vi "CSDB_Config.apply mapping.vi"(1 "Enum":enum16{"i 2 BP", "BP 2 i", "get"}(ring), 2 "ClassName":string, 3 "AttributeNamesIn":string[](array[string]), 4 "Values in":string[][](array[string]), 5 "error in (no error)":errorcluster) -> (17 "AttributeNames out":string[](array[string]), 18 "Values out":string[][](array[string]), 19 "error out":errorcluster)   [LabVIEW 2014, in "CSDB_Config.lvlib"]
doc: "hm..."
uses:
  CSDB_Config.lvlib
  <vilib>/Utility/config.llb/Read Key (String).vi
  <vilib>/Utility/config.llb/NI_LVConfig.lvlib
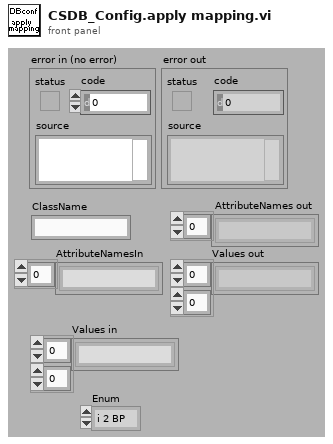
[diagram p1: front panel]
types:
  T1 = typedef "NI_LVConfig.lvlib/Config Data RefNum.ctl" = refnum<k1>
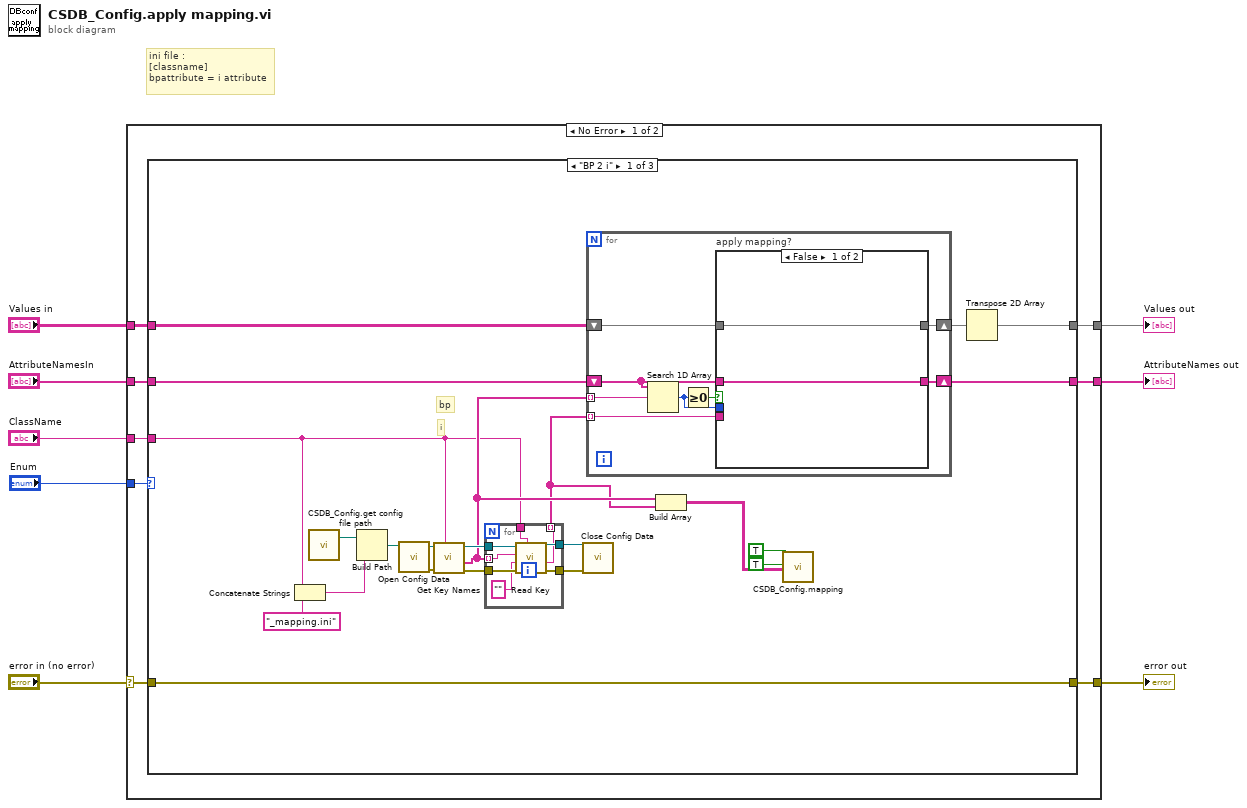
[diagram p0: block diagram]
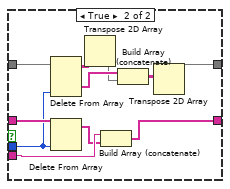
[diagram p2: hidden frame]
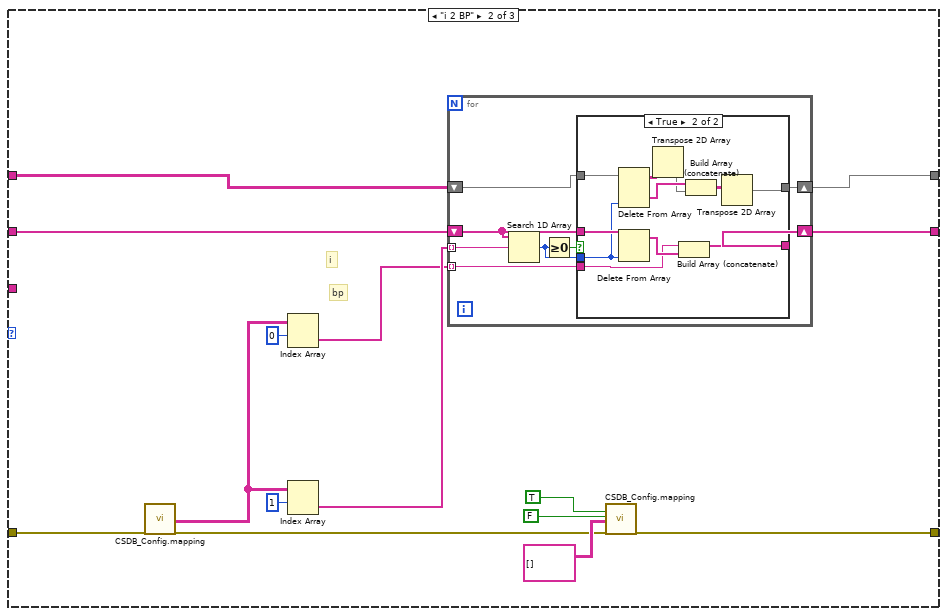
[diagram p3: hidden frame]
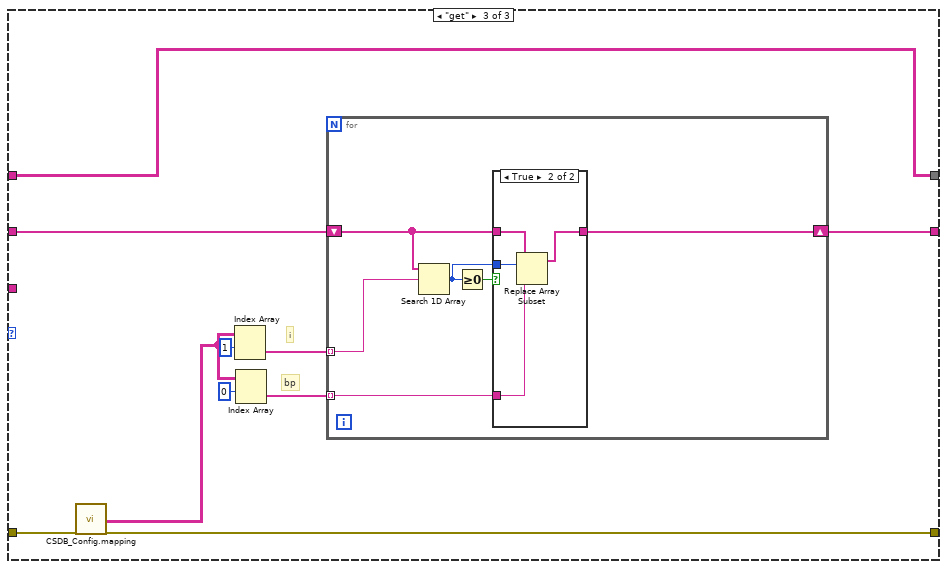
[diagram p5: hidden frame]
diagram:
  # "ini file :\n[classname]\nbpattribute = i attribute"
  n1 = case shown="No Error" "error in (no error)" {
    selector: "error in (no error)" -> [w9 w127]
    tunnel: [w16 w127] -> w8
    tunnel: "ClassName" -> [w15 _]
    tunnel: "AttributeNamesIn" -> [w14 w125]
    tunnel: [w13 w125] -> w5
    tunnel: "Values in" -> [w12 w126]
    tunnel: [w11 w126] -> w3
    tunnel: "Enum" -> [w10 _]
    frame No Error {
      n2 = case shown="\"BP 2 i\"" w10 {
        tunnel: w9 -> [w38 w77 w106]
        tunnel: [w38 w82 w105] -> w16
        tunnel: w15 -> [w18 _ _]
        tunnel: w14 -> [w37 w81 w113]
        tunnel: [w36 w80 w112] -> w13
        tunnel: w12 -> [w35 w79 w111]
        tunnel: [w34 w78 w111] -> w11
        frame "BP 2 i" {
          # "i"
          # "bp"
          n3 = Concatenate Strings(w18, "_mapping.ini" ("name or relative path")) -> (w17:string)
          n4 = call "CSDB_Config.get config file path.vi"() -> ("config file path"=w23:path)  [unwired: 18 in, 1 out]
          n5 = Build Path(base path=w23, name or relative path=w17) -> (appended path=w24:path)
          n6 = call <vilib>:"Open Config Data.vi"("configuration file path"=w24) -> ("error out"=w31:errorcluster, "refnum"=w32:T1)  [unwired: 8 in, 1 out]
          n7 = call <vilib>:"Get Key Names.vi"("section"=w18, "error in (no error)"=w31, "refnum"=w32) -> ("error out"=w29:errorcluster, "key names"=w26:string[], "refnum out"=w30:T1)  [unwired: 5 in, 1 out]
          n8 = for {
            tunnel: w30 -> [w67]
            tunnel: w29 -> [w62]
            tunnel: w18 -> [w66]
            tunnel: w26 -> [w65] mode=indexing
            tunnel: [w64] -> w28
            tunnel: [w63] -> w27
            tunnel: [w60] -> w25 mode=indexing
            n9 = call-poly <vilib>:"Read Key.vi"("section"=w66, "error in (no error)"=w62, "default value"="", "key"=w65, "refnum"=w67) -> ("error out"=w63:errorcluster, "value"=w60:string, "refnum out"=w64:T1)  [unwired: 3 in, 1 out]
          }
          n10 = call <vilib>:"Close Config Data.vi"("error in (no error)"=w27, "refnum"=w28) -> ()  [unwired: 8 in, 2 out]
          n11 = for {
            tunnel: w26 -> [w41] mode=indexing
            tunnel: w25 -> [w42] mode=indexing
            shift-right: [w43] -> w36
            shift-left: w37 -> [w45]
            shift-right: [w39] -> w33
            shift-left: w35 -> [w40]
            n12 = Search 1D Array(1D array=w45, element=w41) -> (index of element=w44:i32)  [unwired: 1 in]
            n13 = Greater Or Equal To 0?(x=w44) -> (x >= 0?=w46:bool)
            n14 = case "apply mapping?" shown="False" w46 {
              tunnel: w45 -> [w48 w59]
              tunnel: w44 -> [_ w56]
              tunnel: w42 -> [_ w54]
              tunnel: [w48 w58] -> w43
              tunnel: w40 -> [w47 w57]
              tunnel: [w47 w55] -> w39
              frame False {
              }
              frame True {
                n15 = Delete From Array(array=w57, index (col)=w56) -> (deleted portion=w52:string[], array with subset deleted=w50:string[][])  [unwired: 2 in]
                n16 = Delete From Array(array=w59, index=w56) -> (array with subset deleted=w53:string[])  [unwired: 1 in, 1 out]
                n17 = Transpose 2D Array(2D array=w50) -> (transposed array=w49:string[][])
                n18 = Build Array (concatenate)(w54, w53) -> (w58:string[])
                n19 = Build Array (concatenate)(w52, w49) -> (w51:string[][])
                n20 = Transpose 2D Array(2D array=w51) -> (transposed array=w55:string[][])
              }
            }
          }
          n21 = Build Array(w26, w25) -> (w22:string[][])
          n22 = call "CSDB_Config.mapping.vi"("setMapping"=TRUE, "useMapping"=TRUE, "mapping"=w22) -> ()  [unwired: 14 in, 3 out]
          n23 = Transpose 2D Array(2D array=w33) -> (transposed array=w34:string[][])
        }
        frame "i 2 BP" {
          # "i"
          # "bp"
          n24 = call "CSDB_Config.mapping.vi"("error in (no error)"=w77) -> ("mapping out"=w71:string[][], "error out"=w70:errorcluster)  [unwired: 16 in, 1 out]
          n25 = Index Array(array=w71, index (row)=0) -> (element=w73:string[])  [unwired: 1 in]
          n26 = Index Array(array=w71, index (row)=1) -> (element=w74:string[])  [unwired: 1 in]
          n27 = for {
            tunnel: w74 -> [w85] mode=indexing
            tunnel: w73 -> [w86] mode=indexing
            shift-right: [w87] -> w80
            shift-left: w81 -> [w89]
            shift-right: [w83] -> w78
            shift-left: w79 -> [w84]
            n28 = Search 1D Array(1D array=w89, element=w85) -> (index of element=w88:i32)  [unwired: 1 in]
            n29 = Greater Or Equal To 0?(x=w88) -> (x >= 0?=w90:bool)
            n30 = case shown="True" w90 {
              tunnel: w89 -> [w92 w103]
              tunnel: w88 -> [_ w97]
              tunnel: w86 -> [_ w100]
              tunnel: [w92 w102] -> w87
              tunnel: w84 -> [w91 w99]
              tunnel: [w91 w95] -> w83
              frame False {
              }
              frame True {
                n31 = Delete From Array(array=w99, index (col)=w97) -> (deleted portion=w98:string[], array with subset deleted=w94:string[][])  [unwired: 2 in]
                n32 = Delete From Array(array=w103, index=w97) -> (array with subset deleted=w101:string[])  [unwired: 1 in, 1 out]
                n33 = Transpose 2D Array(2D array=w94) -> (transposed array=w93:string[][])
                n34 = Build Array (concatenate)(w100, w101) -> (w102:string[])
                n35 = Build Array (concatenate)(w98, w93) -> (w96:string[][])
                n36 = Transpose 2D Array(2D array=w96) -> (transposed array=w95:string[][])
              }
            }
          }
          n37 = call "CSDB_Config.mapping.vi"("setMapping"=TRUE, "useMapping"=FALSE, "mapping"=string[][] [], "error in (no error)"=w70) -> ("error out"=w82:errorcluster)  [unwired: 13 in, 2 out]
        }
        frame "get" {
          # "i"
          # "bp"
          n38 = call "CSDB_Config.mapping.vi"("error in (no error)"=w106) -> ("mapping out"=w104:string[][], "error out"=w105:errorcluster)  [unwired: 16 in, 1 out]
          n39 = Index Array(array=w104, index (row)=1 ("disabled index (col)")) -> (element=w110:string[])  [unwired: 1 in]
          n40 = Index Array(array=w104, index (row)=0 ("disabled index (col)")) -> (element=w107:string[])  [unwired: 1 in]
          n41 = for {
            tunnel: w110 -> [w119] mode=indexing
            tunnel: w107 -> [w115] mode=indexing
            shift-right: [w114] -> w112
            shift-left: w113 -> [w117]
            n42 = Search 1D Array(1D array=w117, element=w119) -> (index of element=w116:i32)  [unwired: 1 in]
            n43 = Greater Or Equal To 0?(x=w116) -> (x >= 0?=w118:bool)
            n44 = case shown="True" w118 {
              tunnel: w117 -> [w120 w124]
              tunnel: w116 -> [_ w123]
              tunnel: w115 -> [_ w122]
              tunnel: [w120 w121] -> w114
              frame False {
              }
              frame True {
                n45 = Replace Array Subset(array=w124, new element=w122, index=w123) -> (w121:string[])
              }
            }
          }
        }
      }
    }
    frame Error {
    }
  }
  "error out" <- w8
  "AttributeNames out" <- w5
  "Values out" <- w3
